vi "Read Joystick.vi"(8 "Joystick Deadbanded Value (default of 0.1)":dbl, 11 "Joystick L 1 DevRef":T1) -> (1 "Joystick L 2 X Axis":dbl, 2 "Joystick L 1 Y Axis":dbl, 3 "Joystick L 1 X Axis":dbl)   [LabVIEW 2014]
uses:
  <vilib>/Rock Robotics/WPI/Joystick/WPI_JoystickDevRef.ctl
  <vilib>/Rock Robotics/WPI/Joystick/WPI_JoystickDeviceEnum.ctl
  Global Variables.vi
  <vilib>/Rock Robotics/WPI/Joystick/WPI_JoystickGetSetRefNum.vi
panel:
  out "Buttons":bool[](array[boolean])
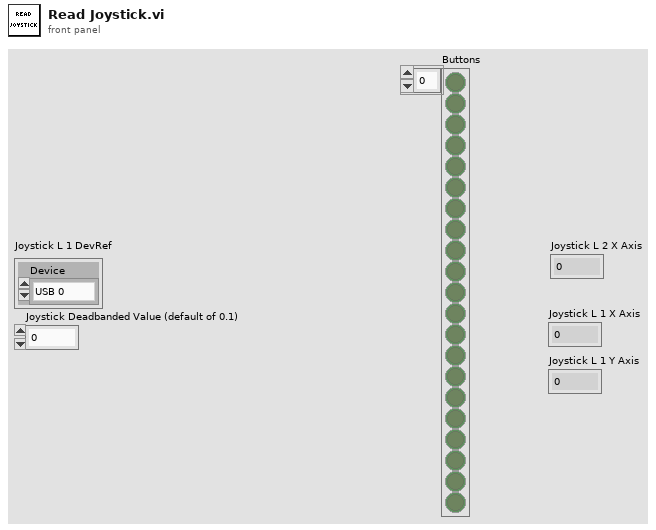
[diagram p1: front panel]
types:
  T1 = typedef "WPI_JoystickDevRef.ctl" = cluster{"Device":T2}
  T2 = typedef "WPI_JoystickDeviceEnum.ctl" = enum16{"USB 0", "USB 1", "USB 2", "USB 3", "USB 4", "USB 5"}
  T3 = cluster{"Buttons[0]":bool, "Buttons[1]":bool, "Buttons[2]":bool, "Buttons[3]":bool, "Buttons[4]":bool, "Buttons[5]":bool, "Buttons[6]":bool, "Buttons[7]":bool, "Buttons[8]":bool}
  T4 = cluster{"Axes[0]":dbl, "Axes[1]":dbl, "Axes[2]":dbl, "Axes[3]":dbl, "Axes[4]":dbl, "Axes[5]":dbl, "Axes[6]":dbl, "Axes[7]":dbl, "Axes[8]":dbl}
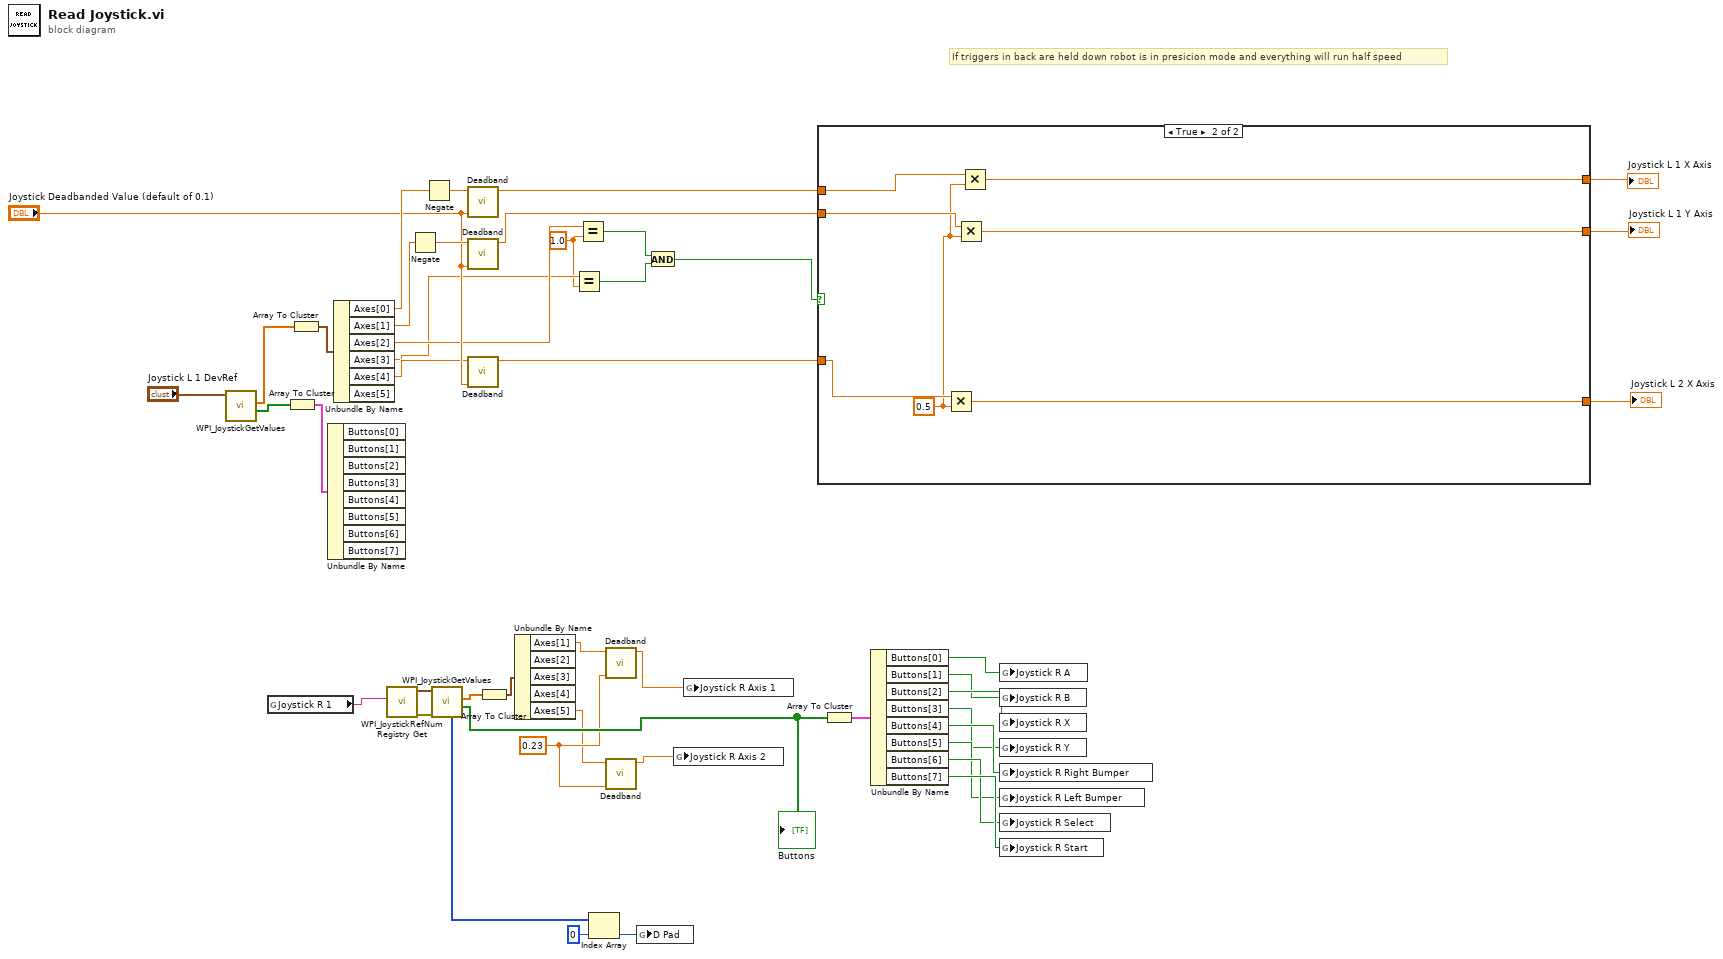
[diagram p0: block diagram]
diagram:
  w16 = 1.0 ("y")
  w5 = 0.23 ("Value to Deadband (default of 0.1)")
  # "If triggers in back are held down robot is in presicion mode and everything will run half speed"
  n1 = call <vilib>:"WPI_JoystickGetValues.vi"("JoystickDevRef"="Joystick L 1 DevRef") -> ("Buttons"=w43:bool[], "Axes"=w45:dbl[])  [unwired: 6 in, 3 out]
  n2 = global read "Global Variables.vi" "Joystick R 1"() -> (w34:string)
  n3 = Array To Cluster(array=w43) -> (cluster=w42:T3)
  n4 = Array To Cluster(array=w45) -> (cluster=w44:T4)
  n5 = Unbundle By Name(w42) -> ()  [unwired: 8 out]
  n6 = Unbundle By Name(w44) -> ("Axes[0]"=w41:dbl, "Axes[1]"=w38:dbl, "Axes[2]"=w18:dbl, "Axes[3]"=w17:dbl, "Axes[4]"=w19:dbl)  [unwired: 1 out]
  n7 = call <vilib>:"WPI_JoystickRefNum Registry Get.vi"("refnum name"=w34) -> ("error out"=w33:errorcluster, "JoystickDevRef"=w32:T1)  [unwired: 9 in]
  n8 = Negate(x=w38) -> (-x=w39:dbl)
  n9 = Negate(x=w41) -> (-x=w40:dbl)
  n10 = call <vilib>:"WPI_JoystickGetValues.vi"("error in (no error)"=w33, "JoystickDevRef"=w32) -> ("Buttons"=w21:bool[], "Axes"=w35:dbl[], "POVs"=w3:i16[])  [unwired: 5 in, 2 out]
  "Buttons" <- w21
  n11 = call "Deadband.vi"("Value to Deadband (default of 0.1)"="Joystick Deadbanded Value (default of 0.1)", "Value"=w40) -> ("Deadbanded Value"=w10:dbl)  [unwired: 9 in]
  n12 = call "Deadband.vi"("Value to Deadband (default of 0.1)"="Joystick Deadbanded Value (default of 0.1)", "Value"=w39) -> ("Deadbanded Value"=w11:dbl)  [unwired: 9 in]
  n13 = call "Deadband.vi"("Value to Deadband (default of 0.1)"="Joystick Deadbanded Value (default of 0.1)", "Value"=w19) -> ("Deadbanded Value"=w12:dbl)  [unwired: 9 in]
  n14 = Array To Cluster(array=w35) -> (cluster=w36:T4)
  n15 = Unbundle By Name(w36) -> ("Axes[1]"=w31:dbl, "Axes[5]"=w4:dbl)  [unwired: 3 out]
  n16 = Equal?(x=w17, y=w16) -> (x = y?=w14:bool)
  n17 = Equal?(x=w18, y=w16) -> (x = y?=w15:bool)
  n18 = Index Array(array=w3, index=0) -> (element=w1:i16)
  n19 = call "Deadband.vi"("Value to Deadband (default of 0.1)"=w5, "Value"=w31) -> ("Deadbanded Value"=w30:dbl)  [unwired: 9 in]
  n20 = call "Deadband.vi"("Value to Deadband (default of 0.1)"=w5, "Value"=w4) -> ("Deadbanded Value"=w6:dbl)  [unwired: 9 in]
  n21 = global write "Global Variables.vi" "D Pad"(w1) -> ()
  n22 = And(x=w15, y=w14) -> (x .and. y?=w13:bool)
  n23 = global write "Global Variables.vi" "Joystick R Axis 2"(w6) -> ()
  n24 = global write "Global Variables.vi" "Joystick R Axis 1"(w30) -> ()
  n25 = case shown="True" w13 {
    tunnel: w12 -> [w47 w56]
    tunnel: w11 -> [w48 w55]
    tunnel: w10 -> [w49 w53]
    tunnel: [w49 w52] -> w9
    tunnel: [w48 w51] -> w8
    tunnel: [w47 w50] -> w7
    frame False {
    }
    frame True {
      w54 = 0.5 ("y")
      n26 = Multiply(x=w56, y=w54) -> (x*y=w50:dbl)
      n27 = Multiply(x=w55, y=w54) -> (x*y=w51:dbl)
      n28 = Multiply(x=w53, y=w54) -> (x*y=w52:dbl)
    }
  }
  "Joystick L 1 Y Axis" <- w8
  "Joystick L 1 X Axis" <- w9
  "Joystick L 2 X Axis" <- w7
  n29 = Array To Cluster(array=w21) -> (cluster=w22:T3)
  n30 = Unbundle By Name(w22) -> ("Buttons[0]"=w20:bool, "Buttons[1]"=w23:bool, "Buttons[2]"=w24:bool, "Buttons[3]"=w25:bool, "Buttons[4]"=w26:bool, "Buttons[5]"=w27:bool, "Buttons[6]"=w28:bool, "Buttons[7]"=w29:bool)
  n31 = global write "Global Variables.vi" "Joystick R A"(w20) -> ()
  n32 = global write "Global Variables.vi" "Joystick R B"(w23) -> ()
  n33 = global write "Global Variables.vi" "Joystick R X"(w24) -> ()
  n34 = global write "Global Variables.vi" "Joystick R Y"(w25) -> ()
  n35 = global write "Global Variables.vi" "Joystick R Right Bumper"(w26) -> ()
  n36 = global write "Global Variables.vi" "Joystick R Left Bumper"(w27) -> ()
  n37 = global write "Global Variables.vi" "Joystick R Select"(w28) -> ()
  n38 = global write "Global Variables.vi" "Joystick R Start"(w29) -> ()
